vi "1 Ball Left Hot Half.vi"(1 "Run?":bool) -> (0 "Done?":bool)   [LabVIEW 2013]
uses:
  Globals/Homes.vi
  Globals/Useful Values.vi
panel:
  out "Sum":dbl
  out "Ready for Vision?":bool
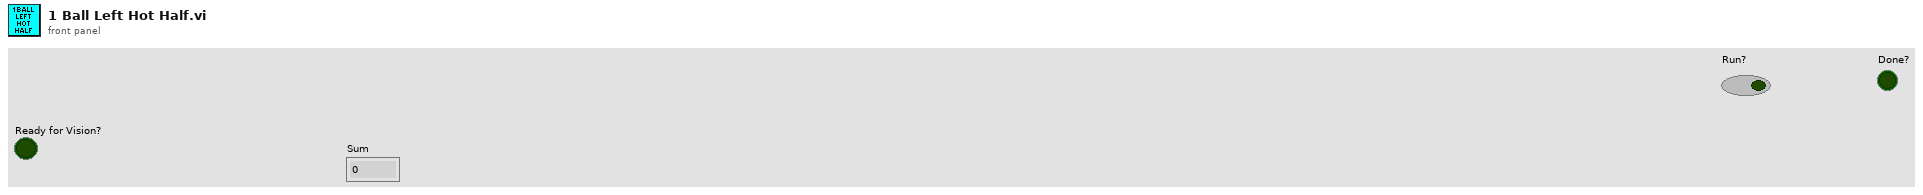
[diagram p1: front panel]
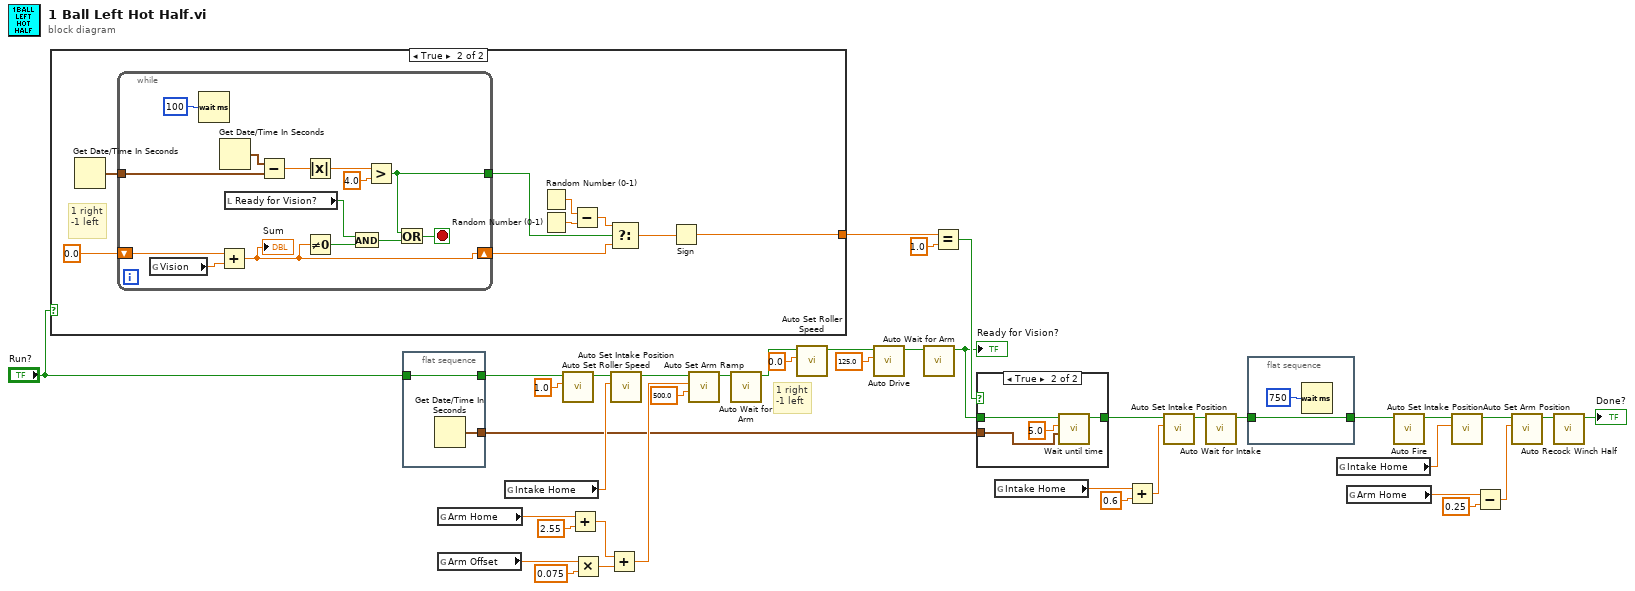
[diagram p0: block diagram]
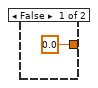
[diagram p3: hidden frame]
diagram:
  # "1 right\n-1 left"
  n1 = case shown="True" "Run?" {
    tunnel: [0.0 w42] -> w8
    frame False {
    }
    frame True {
      # "1 right\n-1 left"
      n2 = Get Date/Time In Seconds() -> (seconds since 1Jan1904=w49:timestamp)
      n3 = while {
        shift-right: [w60] -> w44
        shift-left: 0.0 -> [w63]
        tunnel: w49 -> [w58]
        tunnel: [w51] -> w45
        stop <- w53 stop-if-true
        n4 = global read "Useful Values.vi" "Vision"() -> (w64:dbl)
        n5 = Wait (ms)(milliseconds to wait=u32 100) -> ()  [unwired: 1 out]
        n6 = Add(x=w63, y=w64) -> (x+y=w60:dbl)
        "Sum" <- w60
        n7 = Get Date/Time In Seconds() -> (seconds since 1Jan1904=w57:timestamp)
        n8 = local read "Ready for Vision?"() -> (w61:bool)
        n9 = Subtract(x=w57, y=w58) -> (x-y=w56:dbl)
        n10 = Absolute Value(x=w56) -> (abs(x)=w55:dbl)
        n11 = Not Equal To 0?(x=w60) -> (x != 0?=w59:bool)
        n12 = And(x=w61, y=w59) -> (x .and. y?=w52:bool)
        n13 = Greater?(x=w55, y=4.0) -> (0:w51:bool)
        n14 = Or(x=w51, y=w52) -> (x .or. y?=w53:bool)
      }
      n15 = Random Number (0-1)() -> (number: 0 to 1=w46:dbl)
      n16 = Random Number (0-1)() -> (number: 0 to 1=w47:dbl)
      n17 = Subtract(x=w46, y=w47) -> (x-y=w48:dbl)
      n18 = Select(t=w48, s=w45, f=w44) -> (s? t:f=w43:dbl)
      n19 = Sign(1:w43) -> (0:w42:dbl)
    }
  }
  n20 = flat-sequence {
    tunnel: [w66] -> w5
    tunnel: "Run?" -> [w66]
    tunnel: [w65] -> w3
    frame #0 {
      n21 = Get Date/Time In Seconds() -> (seconds since 1Jan1904=w65:timestamp)
    }
  }
  n22 = global read "Homes.vi" "Arm Home"() -> (w33:dbl)
  n23 = global read "Useful Values.vi" "Arm Offset"() -> (w23:dbl)
  n24 = global read "Homes.vi" "Intake Home"() -> (w32:dbl)
  n25 = call "Auto Set Roller Speed.vi"("Value"=1.0, "Run?"=w5) -> ("Done"=w17:bool)  [unwired: 9 in]
  n26 = Add(x=w33, y=2.55) -> (x+y=w22:dbl)
  n27 = Multiply(x=w23, y=0.075) -> (x*y=w25:dbl)
  n28 = Add(x=w22, y=w25) -> (x+y=w19:dbl)
  n29 = call "Auto Set Intake Position.vi"("Intake Position"=w32, "Run?"=w17) -> ("Done"=w16:bool)  [unwired: 9 in]
  n30 = call "Auto Set Arm Ramp.vi"("Time (ms)"=500.0, "Arm Position"=w19, "Run?"=w16) -> ("Done"=w11:bool)  [unwired: 8 in]
  n31 = call "Auto Wait for Arm.vi"("Run?"=w11) -> ("Done"=w10:bool)  [unwired: 10 in]
  n32 = call "Auto Set Roller Speed.vi"("Value"=0.0, "Run?"=w10) -> ("Done"=w9:bool)  [unwired: 9 in]
  n33 = call "Auto Drive.vi"("Amount"=125.0, "Run?"=w9) -> ("Done"=w12:bool)  [unwired: 9 in]
  n34 = call "Auto Wait for Arm.vi"("Run?"=w12) -> ("Done"=w4:bool)  [unwired: 10 in]
  "Ready for Vision?" <- w4
  n35 = Equal?(x=w8, y=1.0) -> (x = y?=w6:bool)
  n36 = case shown="True" w6 {
    tunnel: w4 -> [w67 w71]
    tunnel: w3 -> [_ w69]
    tunnel: [w67 w68] -> w2
    frame False {
    }
    frame True {
      n37 = call "Wait until time.vi"("Initial Time"=w69, "Time to wait for"=5.0, "Run?"=w71) -> ("Done"=w68:bool)  [unwired: 8 in]
    }
  }
  n38 = global read "Homes.vi" "Intake Home"() -> (w34:dbl)
  n39 = Add(x=w34, y=0.6) -> (x+y=w38:dbl)
  n40 = call "Auto Set Intake Position.vi"("Intake Position"=w38, "Run?"=w2) -> ("Done"=w15:bool)  [unwired: 9 in]
  n41 = call "Auto Wait for Intake.vi"("Run?"=w15) -> ("Done"=w27:bool)  [unwired: 10 in]
  n42 = flat-sequence {
    tunnel: w27 -> [w72]
    tunnel: [w72] -> w26
    frame #0 {
      n43 = Wait (ms)(milliseconds to wait=u32 750) -> ()  [unwired: 1 out]
    }
  }
  n44 = global read "Homes.vi" "Intake Home"() -> (w31:dbl)
  n45 = global read "Homes.vi" "Arm Home"() -> (w29:dbl)
  n46 = call "Auto Fire.vi"("Run?"=w26) -> ("Done"=w37:bool)  [unwired: 10 in]
  n47 = call "Auto Set Intake Position.vi"("Intake Position"=w31, "Run?"=w37) -> ("Done"=w36:bool)  [unwired: 9 in]
  n48 = Subtract(x=w29, y=0.25) -> (x-y=w30:dbl)
  n49 = call "Auto Set Arm Position.vi"("Arm Position"=w30, "Run?"=w36) -> ("Done"=w14:bool)  [unwired: 9 in]
  n50 = call "Auto Recock Winch Half.vi"("Run?"=w14) -> ("Done"=→"Done?":bool)  [unwired: 10 in]
